vi "APU 1.3 Init.vi"(8 "error in (no error)":errorcluster, 11 "rt Data in":T1 {"Compiled Data"."1.1 APUs"."shared settings"."cycle start" format="%#.15g"; "Compiled Data"."1.0 APUs"."shared settings"."cycle start" format="%#.15g"}) -> (0 "error out":errorcluster, 3 "rt Data out":T1 {"Compiled Data"."1.1 APUs"."shared settings"."cycle start" format="%#.15g"; "Compiled Data"."1.0 APUs"."shared settings"."cycle start" format="%#.15g"})   [LabVIEW 2013, in "Engine Simulation Toolkit Engine.lvlib"]
uses:
  Engine Simulation Toolkit Engine.lvlib
  RT Data.ctl
  Shared/Compiled Data.ctl
  Shared/Engine Init Data.ctl
  Shared/1.0 APU Engine Data.ctl
  Shared/1.0 APU Engine FIFO Idxs.ctl
  Shared/Engine Status Data.ctl
  Shared/1.0 Analog Replay Engine Data.ctl
  Shared/1.0 Analog Replay FIFO Idxs.ctl
  Shared/1.0 Digital Pattern Gen Engine Data.ctl
  Shared/1.0 Digital Pattern Gen FIFO Idxs.ctl
  Shared/1.0 Event Timing Capture Engine Data.ctl
  Shared/1.0 Event Timing Capture FIFO Idxs.ctl
  Shared/1.0 Event Timing Measure Engine Data.ctl
  Shared/1.0 Event Timing Measure FIFO Idxs.ctl
  Shared/1.0 Knock Sensor Engine Data.ctl
  Shared/1.0 Knock Sensor FIFO Idxs.ctl
  Shared/1.0 Knock Cylinder Engine Data.ctl
  Shared/1.0 Knock Cylinder FIFO Idxs.ctl
  Shared/1.0 Directional Speed Engine Data.ctl
  Shared/1.0 Directional Speed FIFO Idxs.ctl
  Shared/1.1 APU Engine Data.ctl
  Shared/1.1 Event Timing Measure Engine Data.ctl
  Shared/1.3 Digital Pattern Gen Engine Data.ctl
  Shared/1.3 Digital Pattern Gen FIFO Idxs.ctl
  Shared/Bitfile EST Version.ctl
  Shared/1.3 APU Engine Data.ctl
  FPGA Refs.ctl
  APU 1.0 Run Refs.ctl
  APU 1.0 Output Ref.ctl
  APU 1.0 Input Ref.ctl
  Analog Replay 1.0 Input Ref.ctl
  Digital Pattern Gen 1.0 Input Ref.ctl
  Event Timing Capture 1.0 Output Ref.ctl
  Event Timing Measure 1.0 Output Ref.ctl
  Knock Cylinder 1.0 Input Ref.ctl
  Knock Sensor 1.0 Input Ref.ctl
  Directional Speed 1.0 Input Ref.ctl
  Digital Pattern Gen 1.3 Run Refs.ctl
  Digital Pattern Gen 1.3 Settings Ref.ctl
  APU 1.3 Shared Settings Ref.ctl
  APU 1.3 Settings Ref.ctl
  APU 1.1 Go Ref.ctl
  <vilib>/NI/LVFPGA Adv Session Resources/OpenByNameSubVI.vi
  <vilib>/rvi/interface/common/dynamic/niFpgaEscapeDelimiterAndNull.vi
  <vilib>/Utility/error.llb/Error Cluster From Error Code.vi
  <vilib>/rvi/interface/common/niFpgaWaitOnOcc.vi
  <vilib>/rvi/errors/niLvFpgaAdjustHostInterfaceError.vi
  <vilib>/FPGAPlugInAG/Dynamic/niLvFpga_Close_Dynamic.vi
  <vilib>/NI/LVFPGA Adv Session Resources/OpenByName.xnode
  <vilib>/rvi/interface/nirviReadWriteControl/nirviReadWriteControl.xnode
  <vilib>/rvi/interface/nirviCloseFPGA/nirviCloseFPGA.xnode
  <vilib>/NI/LVFPGA Adv Session Resources/LVFPGAAdvSessionResources.lvlib
  <vilib>/rvi/interface/Simulation/niFpgaSimulationCallBeginRW.vi
  NiFpgaLv.dll
  Shared/Engine Simulation Toolkit Shared.lvlib
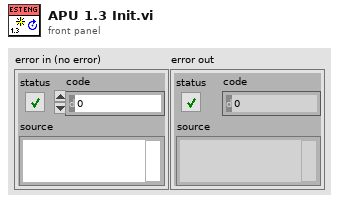
[diagram p1: front panel]
types:
  T1 = typedef "Engine Simulation Toolkit Engine.lvlib/RT Data.ctl" = cluster{"Compiled Data":T2, "FPGA Refs":T27}
  T2 = typedef "Engine Simulation Toolkit Shared.lvlib/Compiled Data.ctl" = cluster{"Init":T3, "1.0 APUs":T4[], "Status":T6, "DevOutFIFO":refnum<k33>, "DevInFIFO":refnum<k33>, "Device Inputs":dbl[], "Device Outputs":dbl[], "Last Device Inputs":dbl[], "1.0 Analog Replays":T7[], "Unused Analog Replays":string[], "1.0 Digital Pattern Gens":T9[], "Unused Digital Pattern Gens":string[], "1.0 Event Captures":T11[], "1.0 Event Measures":T13[], "1.0 Knock Sensors":T15[], "1.0 Knock Cylinders":T17[], "1.0 Directional Speed":T19[], "Unused Directional Sensors":string[], "1.1 APUs":T21[], "1.1 Event Measures":T22[], "1.3 Digital Pattern Gens":T23[], "Bitfile EST Version":T25, "1.3 APUs":T26[]}
  T3 = typedef "Engine Simulation Toolkit Shared.lvlib/Engine Init Data.ctl" = cluster{"CPU":i32, "RIO Address":string, "Decimation":i64, "Priority":i32, "Name":string, "Bitfile Path":path, "Input FIFO Size":i32, "Output FIFO Size":i32}
  T4 = typedef "Engine Simulation Toolkit Shared.lvlib/1.0 APU Engine Data.ctl" = cluster{"register names":cluster{"shared settings":string, "input":string, "settings":string, "output":string}, "shared settings":cluster{"cycle start":fxp<+,2,2>, "crank start":u16, "stuck limit":fxp<+,18,18>}, "settings":cluster{"acceleration":fxp<+,18,-20>, "max cycle":fxp<+,2,2>, "enable accel":bool}, "FIFO indexes":T5, "input":cluster{"desired speed":fxp<+/-,23,2>, "reset":bool}, "degrees of 1 cycle u16":dbl, "degrees of 1 crank u16":dbl}
  T5 = typedef "Engine Simulation Toolkit Shared.lvlib/1.0 APU Engine FIFO Idxs.ctl" = cluster{"inputs":cluster{"desired speed":i32, "reset":i32}, "outputs":cluster{"crank angle":i32, "cycle angle":i32, "actual speed":i32}}
  T6 = typedef "Engine Simulation Toolkit Shared.lvlib/Engine Status Data.ctl" = cluster{"FIFO indexes":cluster{"code":i32, "loop duration":i32, "late count":i32}}
  T7 = typedef "Engine Simulation Toolkit Shared.lvlib/1.0 Analog Replay Engine Data.ctl" = cluster{"register names":cluster{"load input":string, "settings":string, "input":string}, "settings":cluster{"ReverseNegate":bool, "CycleAngle":bool, "SpeedThreshold":fxp<+/-,23,2>, "AOBelowThreshold":i16}, "FIFO indexes":T8, "input":cluster{"Offset":i16, "VScaleSlope":fxp<+,18,6>, "VScaleIntercept":fxp<+/-,18,3>}, "offset convert":dbl, "DAC LUT":i16[], "SE_VScaleIntercept":fxp<+/-,18,3>, "SE_VScaleSlope":fxp<+,18,6>, "VOverride":bool, "ResetVolts":bool}
  T8 = typedef "Engine Simulation Toolkit Shared.lvlib/1.0 Analog Replay FIFO Idxs.ctl" = cluster{"enable voltage":i32, "volt slope":i32, "volt intercept":i32, "offset":i32}
  T9 = typedef "Engine Simulation Toolkit Shared.lvlib/1.0 Digital Pattern Gen Engine Data.ctl" = cluster{"register names":cluster{"load input":string, "settings":string, "input":string}, "settings":cluster{"edge 1":u16, "edge 2":u16, "cycle angle":bool, "enabled":bool, "first falling":bool}, "FIFO indexes":T10, "input":cluster{"Offset":i16}, "offset convert":dbl, "Position LUT":u16[]}
  T10 = typedef "Engine Simulation Toolkit Shared.lvlib/1.0 Digital Pattern Gen FIFO Idxs.ctl" = cluster{"offset":i32}
  T11 = typedef "Engine Simulation Toolkit Shared.lvlib/1.0 Event Timing Capture Engine Data.ctl" = cluster{"register names":cluster{"output":string}, "FIFO indexes":T12, "degrees of 1 u16":dbl, "wrap":bool, "window min":u16, "duration convert":dbl, "default start":dbl, "default end":dbl, "ref angle":dbl}
  T12 = typedef "Engine Simulation Toolkit Shared.lvlib/1.0 Event Timing Capture FIFO Idxs.ctl" = cluster{"start angle":i32, "end angle":i32, "duration":i32}
  T13 = typedef "Engine Simulation Toolkit Shared.lvlib/1.0 Event Timing Measure Engine Data.ctl" = cluster{"register names":cluster{"settings":string, "output":string}, "settings":cluster{"max":u16, "min":u16, "active high":bool, "wrap":bool, "full window":bool}, "FIFO indexes":T14}
  T14 = typedef "Engine Simulation Toolkit Shared.lvlib/1.0 Event Timing Measure FIFO Idxs.ctl" = cluster{"stuck active":i32, "win all active":i32, "win orph start":i32, "win orph end":i32}
  T15 = typedef "Engine Simulation Toolkit Shared.lvlib/1.0 Knock Sensor Engine Data.ctl" = cluster{"register names":cluster{"settings":string, "input":string}, "settings":cluster{"low freq (periods/tick)":fxp<+,32,0>, "high freq (periods/tick)":fxp<+,32,0>, "duration (1.25MHz tics)":fxp<+,18,18>, "low freq speed slope":fxp<+,16,-3>, "low freq speed intercept":fxp<+,10,-10>, "low freq by speed":bool}, "DAC multiplier":dbl, "FIFO indexes":T16, "input":cluster{"low freq scaler":fxp<+,10,0>}}
  T16 = typedef "Engine Simulation Toolkit Shared.lvlib/1.0 Knock Sensor FIFO Idxs.ctl" = cluster{"amp":i32}
  T17 = typedef "Engine Simulation Toolkit Shared.lvlib/1.0 Knock Cylinder Engine Data.ctl" = cluster{"register names":cluster{"settings":string, "input":string}, "settings":cluster{"seed":u16, "reset":bool}, "input":cluster{"probability compare":u16, "high freq scaler":fxp<+,10,0>, "trigger position":u16}, "DAC multiplier":dbl, "FIFO indexes":T18, "Angle multiplier":dbl}
  T18 = typedef "Engine Simulation Toolkit Shared.lvlib/1.0 Knock Cylinder FIFO Idxs.ctl" = cluster{"prob":i32, "amp":i32, "pos":i32}
  T19 = typedef "Engine Simulation Toolkit Shared.lvlib/1.0 Directional Speed Engine Data.ctl" = cluster{"register names":cluster{"settings":string, "input":string, "load input":string}, "settings":cluster{"Upper Value":u16, "Lower Value":u16, "Upper Index":fxp<+,10,10>, "Lower Index":fxp<+,10,10>, "Enabled":bool}, "input":cluster{"td (tics)":u16, "tf (tics)":u16, "tr (tics)":u16}, "FIFO indexes":T20, "Tooth Centers LUT":u16[]}
  T20 = typedef "Engine Simulation Toolkit Shared.lvlib/1.0 Directional Speed FIFO Idxs.ctl" = cluster{"td":i32, "tf":i32, "tr":i32}
  T21 = typedef "Engine Simulation Toolkit Shared.lvlib/1.1 APU Engine Data.ctl" = cluster{"register names":cluster{"shared settings":string, "input":string, "settings":string, "output":string, "go":string}, "shared settings":cluster{"cycle start":fxp<+,2,2>, "crank start":u16, "stuck limit":fxp<+,18,18>}, "settings":cluster{"acceleration":fxp<+,18,-20>, "max cycle":fxp<+,2,2>, "enable accel":bool}, "FIFO indexes":T5, "input":cluster{"desired speed":fxp<+/-,23,2>, "reset":bool}, "degrees of 1 cycle u16":dbl, "degrees of 1 crank u16":dbl}
  T22 = typedef "Engine Simulation Toolkit Shared.lvlib/1.1 Event Timing Measure Engine Data.ctl" = cluster{"register names":cluster{"settings":string, "output":string}, "settings":cluster{"max":u16, "min":u16, "active high":bool, "wrap":bool}, "FIFO indexes":T14}
  T23 = typedef "Engine Simulation Toolkit Shared.lvlib/1.3 Digital Pattern Gen Engine Data.ctl" = cluster{"register names":cluster{"load input":string, "settings":string, "input":string}, "settings":cluster{"edge 1":u16, "edge 2":u16, "cycle angle":bool, "enabled":bool, "first falling":bool, "fault":bool, "fault wrap":bool, "fault value":bool, "fault count":fxp<+,4,4>, "use fault count":bool}, "FIFO indexes":T24, "input":cluster{"Offset":i16}, "deg to u16 scale":dbl, "Position LUT":u16[], "# of teeth":i16, "max angle":dbl}
  T24 = typedef "Engine Simulation Toolkit Shared.lvlib/1.3 Digital Pattern Gen FIFO Idxs.ctl" = cluster{"offset":i32, "command":i32, "rotations":i32, "start angle":i32, "stop angle":i32, "tooth to rem":i32, "trigger":i32, "valid":i32}
  T25 = typedef "Engine Simulation Toolkit Shared.lvlib/Bitfile EST Version.ctl" = enum16{"1.0", "1.1", "1.2", "1.3"}
  T26 = typedef "Engine Simulation Toolkit Shared.lvlib/1.3 APU Engine Data.ctl" = cluster{"register names":cluster{"shared settings":string, "input":string, "settings":string, "output":string, "go":string}, "shared settings":cluster{"start":fxp<+,17,17>, "stuck limit":fxp<+,18,18>}, "settings":cluster{"acceleration":fxp<+,18,-20>, "enable accel":bool}, "FIFO indexes":T5, "input":cluster{"desired speed":fxp<+/-,23,2>, "reset":bool}, "degrees of 1 cycle u16":dbl, "degrees of 1 crank u16":dbl}
  T27 = typedef "Engine Simulation Toolkit Engine.lvlib/FPGA Refs.ctl" = cluster{"1.0 APUs":T28[], "FPGA ref":refnum<k20>, "1.0 Analog Replays":T31[], "1.0 Dig Pat Gens":T32[], "1.0 Event Captures":T33[], "1.0 Event Measures":T34[], "1.0 Knock Cylinders":T35[], "1.0 Knock Sensors":T36[], "1.0 Directional Speed Sensors":T37[], "1.3 Dig Pat Gens":T38[]}
  T28 = typedef "Engine Simulation Toolkit Engine.lvlib/APU 1.0 Run Refs.ctl" = cluster{"output reference":T29, "input reference":T30}
  T29 = typedef "Engine Simulation Toolkit Engine.lvlib/APU 1.0 Output Ref.ctl" = refnum<k20>
  T30 = typedef "Engine Simulation Toolkit Engine.lvlib/APU 1.0 Input Ref.ctl" = refnum<k20>
  T31 = typedef "Engine Simulation Toolkit Engine.lvlib/Analog Replay 1.0 Input Ref.ctl" = refnum<k20>
  T32 = typedef "Engine Simulation Toolkit Engine.lvlib/Digital Pattern Gen 1.0 Input Ref.ctl" = refnum<k20>
  T33 = typedef "Engine Simulation Toolkit Engine.lvlib/Event Timing Capture 1.0 Output Ref.ctl" = refnum<k20>
  T34 = typedef "Engine Simulation Toolkit Engine.lvlib/Event Timing Measure 1.0 Output Ref.ctl" = refnum<k20>
  T35 = typedef "Engine Simulation Toolkit Engine.lvlib/Knock Cylinder 1.0 Input Ref.ctl" = refnum<k20>
  T36 = typedef "Engine Simulation Toolkit Engine.lvlib/Knock Sensor 1.0 Input Ref.ctl" = refnum<k20>
  T37 = typedef "Engine Simulation Toolkit Engine.lvlib/Directional Speed 1.0 Input Ref.ctl" = refnum<k20>
  T38 = typedef "Engine Simulation Toolkit Engine.lvlib/Digital Pattern Gen 1.3 Run Refs.ctl" = cluster{"input":T32, "settings":T39}
  T39 = typedef "Engine Simulation Toolkit Engine.lvlib/Digital Pattern Gen 1.3 Settings Ref.ctl" = refnum<k20>
  T40 = typedef "Engine Simulation Toolkit Engine.lvlib/APU 1.1 Go Ref.ctl" = refnum<k20>
  T41 = typedef "Engine Simulation Toolkit Engine.lvlib/APU 1.3 Settings Ref.ctl" = refnum<k20>
  T42 = typedef "Engine Simulation Toolkit Engine.lvlib/APU 1.3 Shared Settings Ref.ctl" = refnum<k20>
  T43 = cluster{"Name":string, "Depth":u32, "Write? (Deprecated:Use Implementation)":bool, "Physical Channel":u32, "Base Address":u32, "Data Width":u32, "Data Type":enum32{"Boolean", "I8", "I16", "I32", "I64", "U8", "U16", "U32", "U64", "FXP", "CustomControl", "SGL"}, "FXP Properties":variant, "Write Window Address":u32, "Implementation":enum16{"niFpgaTargetToHost", "niFpgaHostToTarget", "niFpgaPeerToPeerWriter", "niFpgaPeerToPeerReader", "niCoreTargetToHost", "niCoreHostToTarget"}, "Control Set":u32}[]
  T44 = cluster{"Name":string, "type":variant, "indicator?":bool}[]
  T45 = cluster{"desired speed":fxp<+/-,23,2>, "reset":bool}
  T46 = cluster{"acceleration":fxp<+,18,-20>, "enable accel":bool}
  T47 = cluster{"start":fxp<+,17,17>, "stuck limit":fxp<+,18,18>}
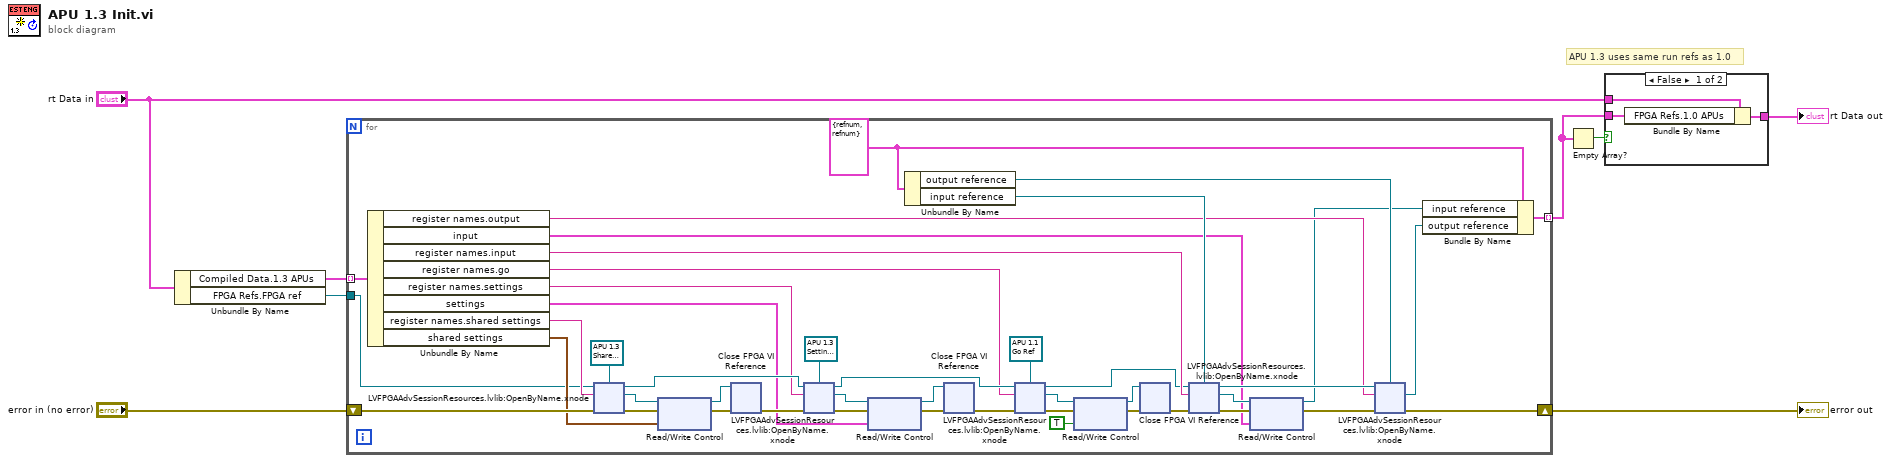
[diagram p0: block diagram]
diagram:
  # "APU 1.3 uses same run refs as 1.0"
  n1 = Unbundle By Name("rt Data in") -> ("Compiled Data.1.3 APUs"=w5:T26[], "FPGA Refs.FPGA ref"=w3:refnum<k20>)
  n2 = for {
    shift-right: [w27] -> w7
    shift-left: "error in (no error)" -> [w52]
    tunnel: w5 -> [w50] mode=indexing
    tunnel: [w34] -> w1 mode=indexing
    tunnel: w3 -> [w24]
    w33 = T28 {"output reference"=refnum, "input reference"=refnum} ("1.0.0 APU Run Refs")
    n3 = Unbundle By Name(w50) -> ("register names.output"=w25:string, "input"=w19:T45, "register names.input"=w26:string, "register names.go"=w15:string, "register names.settings"=w39:string, "settings"=w38:T46, "register names.shared settings"=w49:string, "shared settings"=w46:T47)
    n4 = xnode "LVFPGAAdvSessionResources.lvlib:OpenByName.xnode"("FPGA VI Reference in"=w24, "Resource name in"=w49, "Single resource reference type in"=T42 refnum ("shared settings"), "Error in"=w52) -> ("Single resource reference out"=w47:T42, "Error out"=w51:errorcluster, "FPGA VI Reference out"=w40:refnum<k20>)
    n5 = xnode "Read/Write Control"("FPGA VI Reference In"=w47, "error in"=w51, "Value"=w46) -> ("FPGA VI Reference Out"=w41:T42, "error out"=w43:errorcluster)
    n6 = xnode "Close FPGA VI Reference"("FPGA VI Reference In"=w41, "error in"=w43) -> ("error out"=w42:errorcluster)
    n7 = xnode "LVFPGAAdvSessionResources.lvlib:OpenByName.xnode"("FPGA VI Reference in"=w40, "Resource name in"=w39, "Single resource reference type in"=T41 refnum ("apu settings"), "Error in"=w42) -> ("Single resource reference out"=w45:T41, "Error out"=w44:errorcluster, "FPGA VI Reference out"=w17:refnum<k20>)
    n8 = xnode "Read/Write Control"("FPGA VI Reference In"=w45, "error in"=w44, "Value"=w38) -> ("FPGA VI Reference Out"=w35:T41, "error out"=w36:errorcluster)
    n9 = Unbundle By Name(w33) -> ("output reference"=w30:T29, "input reference"=w29:T30)
    n10 = xnode "Close FPGA VI Reference"("FPGA VI Reference In"=w35, "error in"=w36) -> ("error out"=w31:errorcluster)
    n11 = xnode "LVFPGAAdvSessionResources.lvlib:OpenByName.xnode"("FPGA VI Reference in"=w17, "Resource name in"=w15, "Single resource reference type in"=T40 refnum ("go reference"), "Error in"=w31) -> ("Single resource reference out"=w13:T40, "Error out"=w18:errorcluster, "FPGA VI Reference out"=w12:refnum<k20>)
    n12 = xnode "Read/Write Control"("FPGA VI Reference In"=w13, "error in"=w18, "Value"=TRUE) -> ("FPGA VI Reference Out"=w9:T40, "error out"=w14:errorcluster)
    n13 = xnode "Close FPGA VI Reference"("FPGA VI Reference In"=w9, "error in"=w14) -> ("error out"=w10:errorcluster)
    n14 = xnode "LVFPGAAdvSessionResources.lvlib:OpenByName.xnode"("FPGA VI Reference in"=w12, "Resource name in"=w26, "Single resource reference type in"=w29, "Error in"=w10) -> ("Single resource reference out"=w22:T30, "Error out"=w23:errorcluster, "FPGA VI Reference out"=w32:refnum<k20>)
    n15 = xnode "Read/Write Control"("FPGA VI Reference In"=w22, "error in"=w23, "Value"=w19) -> ("FPGA VI Reference Out"=w21:T30, "error out"=w20:errorcluster)
    n16 = xnode "LVFPGAAdvSessionResources.lvlib:OpenByName.xnode"("FPGA VI Reference in"=w32, "Resource name in"=w25, "Single resource reference type in"=w30, "Error in"=w20) -> ("Single resource reference out"=w28:T29, "Error out"=w27:errorcluster)  [unwired: 1 out]
    n17 = Bundle By Name(cluster=w33, "input reference"=w21, "output reference"=w28) -> (w34:T28)
  }
  "error out" <- w7
  n18 = Empty Array?(array=w1) -> (empty?=w2:bool)
  n19 = case shown="False" w2 {
    tunnel: "rt Data in" -> [w120 w121]
    tunnel: [w119 w121] -> w4
    tunnel: w1 -> [w118 _]
    frame False {
      n20 = Bundle By Name(cluster=w120, "FPGA Refs.1.0 APUs"=w118) -> (w119:T1)
    }
    frame True {
    }
  }
  "rt Data out" <- w4
